vi "PH_Revolver-GUI_6P.set i Attr and start DIM services.vi"(0 "i ref in":refnum<vi>, 5 "error in (no error)":errorcluster) -> (14 "i ref out":refnum<vi>, 16 "i Attributes":T1={"GUI Refs"={"0°"=refnum, "60°"=refnum, "120°"=refnum, "180°"=refnum, "240°"=refnum, "300°"=refnum, "Action"=refnum}, "Revolver Position"=0, "Service ID Position"=-1, "Captions"=[]} {"Revolver Position" items=["unknown", "Position 0", "Position 60", "Position 120", "Position 180", "Position 240", "Position 300", "moving"]}, 19 "error out":errorcluster)   [LabVIEW 2014, in "PH_Revolver-GUI_6P.lvlib"]
doc: "This VI reads the DB special 0 and 1 DB entries which are the axis names and writes them to own attributes. Depending on this, several GUI elements are set."
uses:
  PH_Revolver-GUI_6P.lvlib
  PH_Revolver-GUI_6P.i attribute.ctl
  PH_Revolver-GUI_6P.Position.ctl
  PH_Basics/PH_Common/PH_Common.lvlib
  CS_Core/CSSystem/CSSystemLib/CSSystemLib.lvlib
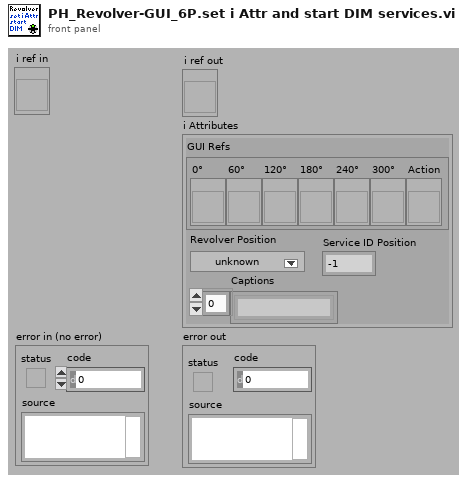
[diagram p1: front panel]
types:
  T1 = typedef "PH_Revolver-GUI_6P.lvlib/PH_Revolver-GUI_6P.i attribute.ctl" = cluster{"GUI Refs":cluster{"0°":refnum<vi>, "60°":refnum<vi>, "120°":refnum<vi>, "180°":refnum<vi>, "240°":refnum<vi>, "300°":refnum<vi>, "Action":refnum<vi>}, "Revolver Position":T2, "Service ID Position":i32, "Captions":string[]}
  T2 = typedef "PH_Revolver-GUI_6P.lvlib/PH_Revolver-GUI_6P.Position.ctl" = u16
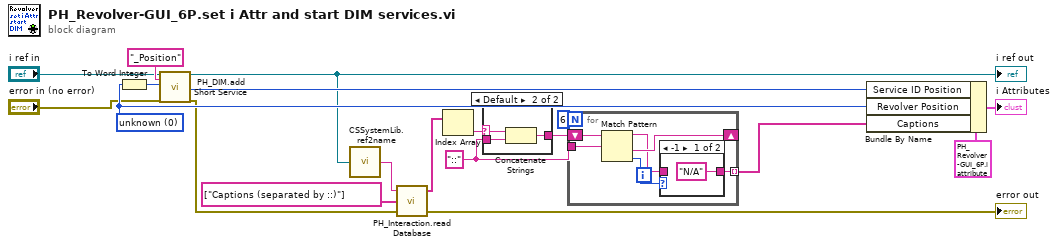
[diagram p0: block diagram]
diagram:
  w10 = "::" ("regular expression")
  w17 = T2 0 items=["unknown", "Position 0", "Position 60", "Position 120", "Position 180", "Position 240", "Position 300", "moving"] ("Revolver Position")
  n1 = To Word Integer(number=w17) -> (16bit integer=w15:i16)
  n2 = call "PH_DIM.add Short Service.vi"("i ref in"="i ref in", "Service Name"="_Position", "Number"=w15, "error in (no error)"="error in (no error)") -> ("i ref out"=w3:refnum<vi>, "Service ID"=w13:i32, "error out"=w5:errorcluster)  [unwired: 13 in]
  "i ref out" <- w3
  n3 = call "CSSystemLib.ref2name.vi"("obj refnum"=w3) -> ("name"=w2:string)
  n4 = call "PH_Interaction.read Database.vi"("error in (no error)"=w5, "Strings to search for"=string[] ["Captions (separated by ::)"] ("Strings to search for in"), "DB Entry to read"=w2) -> ("error out"=→"error out":errorcluster, "Values"=w9:string[])  [unwired: 1 in]
  n5 = Index Array(array=w9) -> (element=w8:string)  [unwired: 1 in]
  n6 = case shown="Default" w8 {
    selector: w8 -> [w20 w23]
    tunnel: [w20 w22] -> w11
    tunnel: w10 -> [_ w21]
    frame "", "N/A" {
    }
    frame Default {
      n7 = Concatenate Strings(w23, w21) -> (w22:string)
    }
  }
  n8 = for {
    N: 6 -> [_]
    shift-right: [w28] -> _
    shift-left: w11 -> [w29]
    tunnel: [w25] -> w7 mode=indexing
    tunnel: w10 -> [w24]
    n9 = Match Pattern(string=w29, regular expression=w24) -> (before substring=w26:string, after substring=w28:string, offset past match=w27:i32)  [unwired: 1 in, 1 out]
    n10 = case shown="-1" w27 {
      tunnel: w26 -> [_ w31]
      tunnel: ["N/A" ("Labels (::-separated)") w31] -> w25
      frame -1 {
      }
      frame Default {
      }
    }
  }
  n11 = Bundle By Name(cluster=T1 {"GUI Refs"={"0°"=refnum, "60°"=refnum, "120°"=refnum, "180°"=refnum, "240°"=refnum, "300°"=refnum, "Action"=refnum}, "Revolver Position"=0, "Service ID Position"=0, "Captions"=[]} ("i attribute"), "Service ID Position"=w13, "Revolver Position"=w17, "Captions"=w7) -> (→"i Attributes":T1)
